vi "Toggle_Pnuematic_State.vi"(1 "Boolean":bool, 2 "Solonoid_In":T1={"DevStatus"={"status"=FALSE, "code"=0, "source"=""}, "Pneumatics Control Module"=0, "Forward Solenoid Channel"=enum."Invalid", "Reverse Solenoid Channel"=enum."Invalid"}) -> (0 "Solenoid_Out":T3)   [LabVIEW 2018]
uses:
  <vilib>/Rock Robotics/WPI/Solenoid/WPI_SolenoidValue.ctl
  <vilib>/Rock Robotics/WPI/Solenoid/WPI_SolenoidDevRef.ctl
  <vilib>/Rock Robotics/WPI/Solenoid/WPI_SolenoidChannel.ctl
  <vilib>/Rock Robotics/WPI/DriverStation/WPI_DriverStationRobotMode2.ctl
  Global_Variables/Robot_Global_Data.vi
  <vilib>/Rock Robotics/WPI/Solenoid/WPI_SolenoidGetEnum.vi
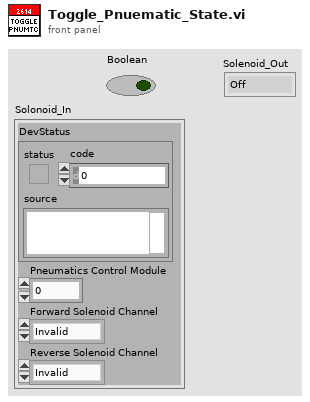
[diagram p1: front panel]
types:
  T1 = typedef "WPI_SolenoidDevRef.ctl" = cluster{"DevStatus":errorcluster, "Pneumatics Control Module":u8, "Forward Solenoid Channel":T2, "Reverse Solenoid Channel":T2}
  T2 = typedef "WPI_SolenoidChannel.ctl" = enum8{"Solenoid 0", "Solenoid 1", "Solenoid 2", "Solenoid 3", "Solenoid 4", "Solenoid 5", "Solenoid 6", "Solenoid 7", "Invalid"}
  T3 = typedef "WPI_SolenoidValue.ctl" = enum16{"Off", "On", "Forward", "Reverse"}
  T4 = typedef "WPI_DriverStationRobotMode2.ctl" = enum16{"Autonomous Disabled", "Autonomous Enabled", "Teleop Disabled", "Teleop Enabled", "Disconnected", "Finish", "Test Disabled", "Test Enabled", "Emergency Stopped"}
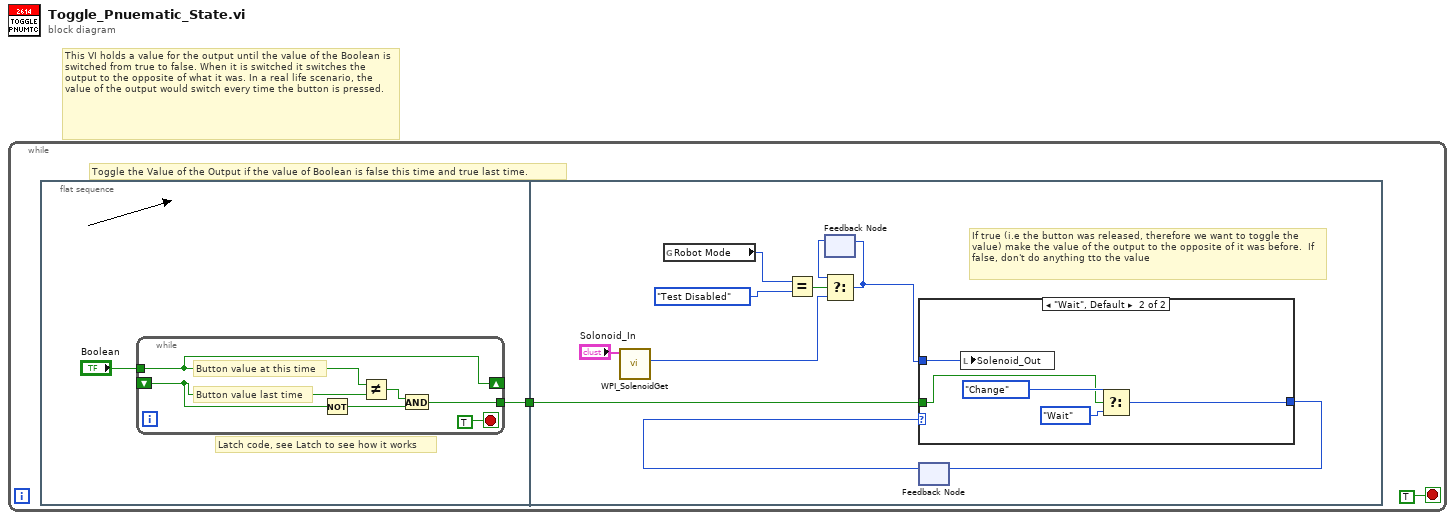
[diagram p0: block diagram]
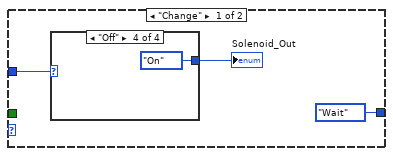
[diagram p2: hidden frame]
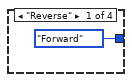
[diagram p3: hidden frame]
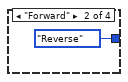
[diagram p4: hidden frame]
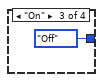
[diagram p5: hidden frame]
diagram:
  # "This VI holds a value for the output until the value of the Boolean is switched from true to false. When it is switched it switches the output to the opposite of what it was. In a real life scenario, the value of the output would switch every time the button is pressed."
  n1 = while {
    stop <- TRUE stop-if-true
    # "Toggle the Value of the Output if the value of Boolean is false this time and true last time."
    n2 = flat-sequence {
      tunnel: [w3] -> w1
      tunnel: w1 -> [w20]
      frame #0 {
        # "Latch code, see Latch to see how it works"
        n3 = while {
          tunnel: [w7] -> w3
          tunnel: "Boolean" -> [w10]
          shift-right: [w10] -> _
          shift-left: _ -> [w6]
          stop <- TRUE ("stop") stop-if-true
          # "Button value last time"
          # "Button value at this time"
          n4 = Not(x=w6) -> (.not. x?=w5:bool)
          n5 = Not Equal?(x=w10, y=w6) -> (x != y?=w8:bool)
          n6 = And(x=w8, y=w5) -> (x .and. y?=w7:bool)
        }
      }
      frame #1 {
        # "If true (i.e the button was released, therefore we want to toggle the value) make the value of the output to the opposite of it was before.  If false, don't do anything tto the value"
        n7 = call-poly <vilib>:"WPI_SolenoidGet.vi"("SolenoidDevRef"="Solonoid_In") -> ("Value"=w13:T3)  [unwired: 8 in, 2 out]
        n8 = global read "Robot_Global_Data.vi" "Robot Mode"() -> (w14:T4)
        n9 = Equal?(x=w14, y=WPI_DriverStationRobotMode2."Test Disabled") -> (x = y?=w16:bool)
        n10 = feedback #1() -> (w11:T3)  [unwired: 1 in]
        n11 = Select(t=w11, s=w16, f=w13) -> (s? t:f=w12:T3)
        n12 = feedback-in #1(w12) -> ()
        n13 = feedback #2() -> (w18:enum16{"Change", "Wait"})  [unwired: 1 in]
        n14 = case shown="\"Wait\", Default" w18 {
          tunnel: w20 -> [_ w31]
          tunnel: [enum16{"Change", "Wait"}."Wait" w30] -> w19
          tunnel: w12 -> [w22 w28]
          frame "Change" {
            n15 = case shown="\"Off\"" w22 {
              tunnel: [WPI_SolenoidValue."Forward" ("Value") WPI_SolenoidValue."Reverse" ("Value") WPI_SolenoidValue."Off" ("Value") WPI_SolenoidValue."On" ("Value")] -> w21
              frame "Reverse" {
              }
              frame "Forward" {
              }
              frame "On" {
              }
              frame "Off" {
              }
            }
            "Solenoid_Out" <- w21
          }
          frame "Wait", Default {
            n16 = local write "Solenoid_Out"(w28) -> ()
            n17 = Select(t=enum16{"Change", "Wait"}."Change", s=w31, f=enum16{"Change", "Wait"}."Wait") -> (s? t:f=w30:enum16{"Change", "Wait"})
          }
        }
        n18 = feedback-in #2(w19) -> ()
      }
    }
  }
